vi "Agilent 34970 EZ Scan.vi"() -> ()   [LabVIEW 2011]
doc: "This Example VI shows how to set up the scan list and then take a measurement. This VI uses the EZ measurement VIs. These VIs offer the quickest and easiest use. However, they do not let you have different types of measurements in the same scan list. For a full description of the three ways to setup and scan using the HP34970A, read the text below.\n\nAlthough this driver only shows Current and Frequency (for simplicity), there are EZ Measurement VIs for all six measurement types.\n\n====================\nSetting up and performing a scan\n====================\nThe HP34970A provides commands for setting up a scan in three ways that differ in their complexity and the amount of control offered:\n\n1. Advanced:\nEvery aspect of the measurement, scan, scan list, and read is put in a different command to allow the greatest flexibility. For example, using the advanced configure VIs, you can set up a scan list consisting of different measurement types on different channels. The \"HP34970A Advanced Scan Example.vi\" demonstrates usage of these VIs.\n\n2. Medium:\nThe instrument also offers a command that wraps up configuring individual channels and the scan list. This is represented in the driver by \"HP34970A Conf EZ.vi\". This driver specifically replaces use of the advanced configure measurement VIs and configure scan list VIs. For more information, refer to the context help for the Conf EZ VI.\n\n3. Easiest:\nThe entire configuration, scan, and read are wrapped up into one command to the instrument. This is provided in this driver as the \"EZ\" VIs, which are in the Data subpalette of the HP34970A's driver palette. The \"HP34970A EZ Scan Example.vi\" demonstrates the EZ VI's usage."
uses:
  <vilib>/Platform/TimedLoop/XDataNode/timing_clust.ctl
  <vilib>/Platform/TimedLoop/XDataNode/nitl_modes.ctl
  <vilib>/Platform/TimedLoop/XDataNode/wakeup.ctl
  <vilib>/addons/database/Connection.llb/DB Tools Open Connec (String).vi
  <vilib>/Platform/TimedLoop/XDataNode/XDataNode.xnode
  <instrlib>/Agilent 34970/Agilent 34970.lvlib
  <vilib>/Platform/TimedLoop/XDataNode/XDNodeRunTimeDep.lvlib
  <vilib>/addons/database/NI_Database_API.lvlib
panel:
  out "timestamp":timestamp
  in  "stop":bool
  in  "Period [s]":i64=10
  out "error out":errorcluster
  out "Temperature \nChannel 101:106 [°C]":dbl[](array[numeric]) format="%.2f"
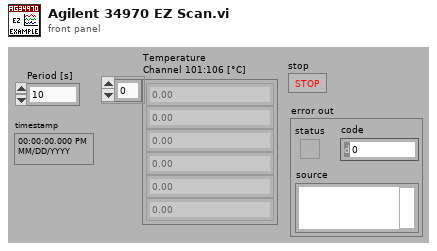
[diagram p1: front panel]
types:
  T1 = cluster{"Timeout Value (10000)":u32, "Baud Rate (57600)":enum16{"1200", "2400", "4800", "9600", "19200", "38400", "57600", "115200"}, "Flow Control (1:XON/XOFF)":enum16{"None", "XON / XOFF", "RTS / CTS", "DTR / DSR"}}
  T2 = typedef "NI_Database_API.lvlib/Conn ObjectReference.ctl" = refnum<k1>
  T3 = typedef "XDNodeRunTimeDep.lvlib/timing_clust.ctl" = cluster{"Expected End [f-1]":u64, "Actual End [f-1]":u64, "Finished Late? [f-1]":bool, "Expected End [i-1]":u64, "Actual End [i-1]":u64, "Finished Late? [i-1]":bool, "Expected Start [i]":u64, "Actual Start [i]":u64, "Expected Start [f]":u64, "Actual Start [f]":u64, "Source Name":string, "Structure Name":string, "Period":i64, "Deadline":i64, "Offset":i64, "Start":i64, "Priority":i32, "Timeout":i32, "Mode":T4, "Wakeup Reason":T5, "Error":errorcluster, "Source Type":string, "Secondary Source Type":string, "Global End Time":u64, "Global Start Time":u64, "Frame Duration":u64, "Iteration Duration":u64, "Assigned CPU":i32, "I/O Scan Engine Mode":u32}
  T4 = typedef "XDNodeRunTimeDep.lvlib/nitl_modes.ctl" = enum32{"No Change", "Process missed periods, maintain original phase", "Discard missed periods, maintain original phase", "Process missed periods, ignore original phase", "Discard missed periods, ignore original phase"}
  T5 = typedef "XDNodeRunTimeDep.lvlib/wakeup.ctl" = enum32{"Normal", "Aborted", "Asynchronous wakeup", "Timing source error", "Timed loop error", "Timeout"}
  T6 = enum16{"Thermocouple", "Thermistor", "RTD", "4-Wire RTD", "Default (Last)"}
  T7 = enum16{"2252", "5000", "10000", "Default (Last)"}
  T8 = enum16{"B", "E", "J", "K", "N", "R", "S", "T", "Default (Last)"}
  T9 = cluster{"Output Array[0]":dbl, "Output Array[1]":dbl, "Output Array[2]":dbl, "Output Array[3]":dbl, "Output Array[4]":dbl, "Output Array[5]":dbl, "Output Array[6]":dbl, "Output Array[7]":dbl, "Output Array[8]":dbl}
  T10 = cluster{"seconds since 1Jan1904":timestamp, "Output Array[0]":dbl}
  T11 = cluster{"seconds since 1Jan1904":timestamp, "Output Array[1]":dbl}
  T12 = cluster{"seconds since 1Jan1904":timestamp, "Output Array[2]":dbl}
  T13 = cluster{"seconds since 1Jan1904":timestamp, "Output Array[3]":dbl}
  T14 = cluster{"seconds since 1Jan1904":timestamp, "Output Array[4]":dbl}
  T15 = cluster{"seconds since 1Jan1904":timestamp, "Output Array[5]":dbl}
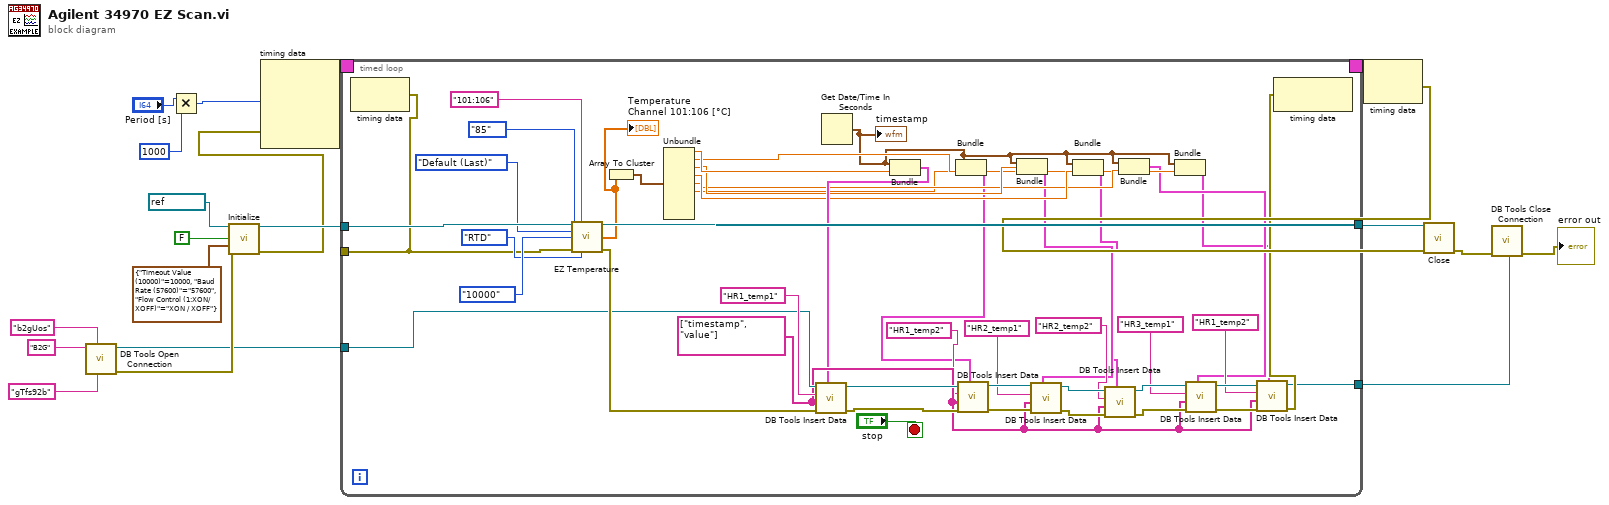
[diagram p0: block diagram]
diagram:
  n1 = call-poly <vilib>:"DB Tools Open Connection.vi"("password"="gTfs92b", "userID"="b2gUos", "connection information"="B2G") -> ("error out"=w5:errorcluster, "connection reference"=w4:T2)  [unwired: 5 in]
  n2 = Multiply(x="Period [s]", y=i64 1000) -> (x*y=w9:i64)
  n3 = call <instrlib>:"Initialize.vi"("VISA Resource Name"=refnum<visa-resource-name> "COM1" ("VISA resource name"), "Reset (T: Reset)"=FALSE ("Reset"), "Serial Port Configuration"=T1 {"Timeout Value (10000)"=10000, "Baud Rate (57600)"=enum."57600", "Flow Control (1:XON/XOFF)"=enum."XON / XOFF"}, "error in (no error)"=w5) -> ("VISA Resource Name Out"=w17:refnum<visa-resource-name>, "error out"=w13:errorcluster)  [unwired: 10 in]
  n4 = node-c288(w9, w13) -> (w15:T3)  [unwired: 2 in]
  n5 = timed-loop {
    timing: w15 -> [_]
    timing-out: [_] -> w14
    tunnel: w17 -> [w65]
    tunnel: [w58] -> _
    tunnel: [w63] -> w16
    tunnel: w4 -> [w52]
    tunnel: [w40] -> w3
    stop <- "stop" stop-if-true
    w39 = string[] ["timestamp", "value"] ("columns")
    n6 = node-c288() -> (w58:errorcluster)  [unwired: 1 in]
    n7 = call <instrlib>:"EZ Temperature.vi"("VISA Resource Name"=w65, "Scan List (empty)"="101:106" ("Channel List"), "Thermocouple Type (8:Def-Last)"=T8."Default (Last)" ("Thermocouple Type"), "Thermistor Type (3:Def-Last)"=T7."10000" ("Thermistor Type"), "RTD Type (2:Default-Last)"=enum16{"85", "91", "Default (Last)"}."85" ("RTD Type"), "error in (no error)"=w58, "Transducer Type (4:Def-Last)"=T6."RTD" ("Transducer Type")) -> ("VISA Resource Name Out"=w63:refnum<visa-resource-name>, "Output Array"=w54:dbl[], "error out"=w55:errorcluster)  [unwired: 6 in]
    "Temperature \nChannel 101:106 [°C]" <- w54
    n8 = Array To Cluster(array=w54) -> (cluster=w53:T9)
    n9 = Unbundle(w53) -> ("Output Array[0]"=w33:dbl, "Output Array[1]"=w31:dbl, "Output Array[2]"=w30:dbl, "Output Array[3]"=w29:dbl, "Output Array[4]"=w27:dbl, "Output Array[5]"=w26:dbl)  [unwired: 3 out]
    n10 = Get Date/Time In Seconds() -> (seconds since 1Jan1904=w28:timestamp)
    "timestamp" <- w28
    n11 = Bundle("seconds since 1Jan1904"=w28, "Output Array[0]"=w33) -> (w32:T10)  [unwired: 1 in]
    n12 = call <vilib>:"DB Tools Insert Data.vi"("data"=w32, "error in (no error)"=w55, "columns"=w39, "table"="HR1_temp1", "connection reference"=w52) -> ("error out"=w51:errorcluster, "connection reference out"=w45:T2)  [unwired: 5 in]
    n13 = Bundle("seconds since 1Jan1904"=w28, "Output Array[1]"=w31) -> (w25:T11)  [unwired: 1 in]
    n14 = call <vilib>:"DB Tools Insert Data.vi"("data"=w25, "error in (no error)"=w51, "columns"=w39, "table"="HR1_temp2", "connection reference"=w45) -> ("error out"=w50:errorcluster, "connection reference out"=w44:T2)  [unwired: 5 in]
    n15 = Bundle("seconds since 1Jan1904"=w28, "Output Array[2]"=w30) -> (w24:T12)  [unwired: 1 in]
    n16 = call <vilib>:"DB Tools Insert Data.vi"("data"=w24, "error in (no error)"=w50, "columns"=w39, "table"="HR2_temp1", "connection reference"=w44) -> ("error out"=w49:errorcluster, "connection reference out"=w43:T2)  [unwired: 5 in]
    n17 = Bundle("seconds since 1Jan1904"=w28, "Output Array[3]"=w29) -> (w23:T13)  [unwired: 1 in]
    n18 = call <vilib>:"DB Tools Insert Data.vi"("data"=w23, "error in (no error)"=w49, "columns"=w39, "table"="HR2_temp2", "connection reference"=w43) -> ("error out"=w48:errorcluster, "connection reference out"=w42:T2)  [unwired: 5 in]
    n19 = Bundle("seconds since 1Jan1904"=w28, "Output Array[4]"=w27) -> (w22:T14)  [unwired: 1 in]
    n20 = Bundle("seconds since 1Jan1904"=w28, "Output Array[5]"=w26) -> (w21:T15)  [unwired: 1 in]
    n21 = call <vilib>:"DB Tools Insert Data.vi"("data"=w22, "error in (no error)"=w48, "columns"=w39, "table"="HR3_temp1", "connection reference"=w42) -> ("error out"=w47:errorcluster, "connection reference out"=w41:T2)  [unwired: 5 in]
    n22 = call <vilib>:"DB Tools Insert Data.vi"("data"=w21, "error in (no error)"=w47, "columns"=w39, "table"="HR1_temp2", "connection reference"=w41) -> ("error out"=w46:errorcluster, "connection reference out"=w40:T2)  [unwired: 5 in]
    n23 = node-c288(w46) -> ()  [unwired: 1 out]
  }
  n24 = node-c288(w14) -> (w12:errorcluster)
  n25 = call <instrlib>:"Close.vi"("VISA Resource Name"=w16, "error in (no error)"=w12) -> ("error out"=w2:errorcluster)  [unwired: 13 in]
  n26 = call <vilib>:"DB Tools Close Connection.vi"("error in (no error)"=w2, "connection reference"=w3) -> ("error out"=→"error out":errorcluster)  [unwired: 5 in]
